vi "Read Ctl Refnum.vi"(8 "error in (no error)":errorcluster, 11 "String Control in":refnum<class "String Control.lvclass">) -> (0 "error out":errorcluster, 2 "Ctl Refnum":refnum<vi>, 3 "String Control out":refnum<class "String Control.lvclass">)   [LabVIEW 2010, in "String Control.lvclass"]
uses:
  String Control.lvclass
  String Control.lvclass/String Control.ctl
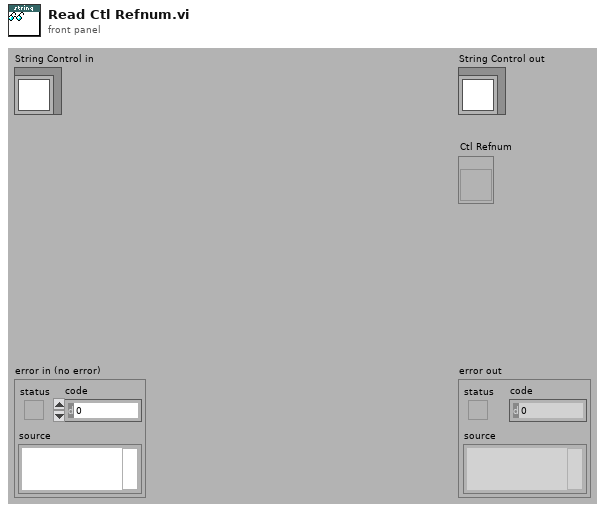
[diagram p1: front panel]
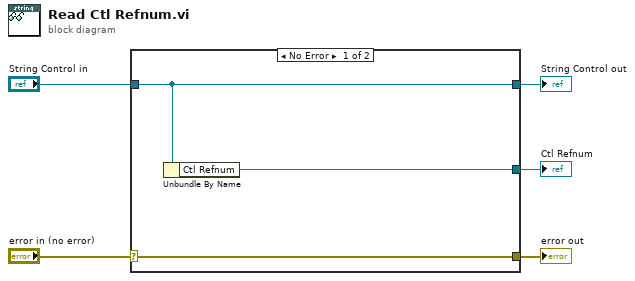
[diagram p0: block diagram]
diagram:
  n1 = case shown="No Error" "error in (no error)" {
    selector: "error in (no error)" -> [w8 w9]
    tunnel: [w8 w9] -> w4
    tunnel: [w7 w10] -> w2
    tunnel: "String Control in" -> [w7 w10]
    tunnel: [w6 _] -> w1
    frame No Error {
      n2 = Unbundle By Name(w7) -> ("Ctl Refnum"=w6:refnum<vi>)
    }
    frame Error {
    }
  }
  "error out" <- w4
  "String Control out" <- w2
  "Ctl Refnum" <- w1
